vi "set-reporting-device.vi"(5 "ttl":i32, 6 "wait for reply (T)":bool=TRUE, 7 "device-name":string, 8 "error in":errorcluster, 9 "period-ms":i32, 10 "measurement-list":string[](array[string]), 11 "Module ID":i32=-1) -> (0 "error out":errorcluster, 1 "timed out?":bool, 2 "ack":bool)   [LabVIEW 2020, in "reporting-device.lvlib"]
doc: "_____\nCreated using DQMH Event Scripter 7.0.1.1316."
uses:
  reporting-device.lvlib
  set-reporting-device Argument--cluster.ctl
  set-reporting-device (Reply Payload)--cluster.ctl
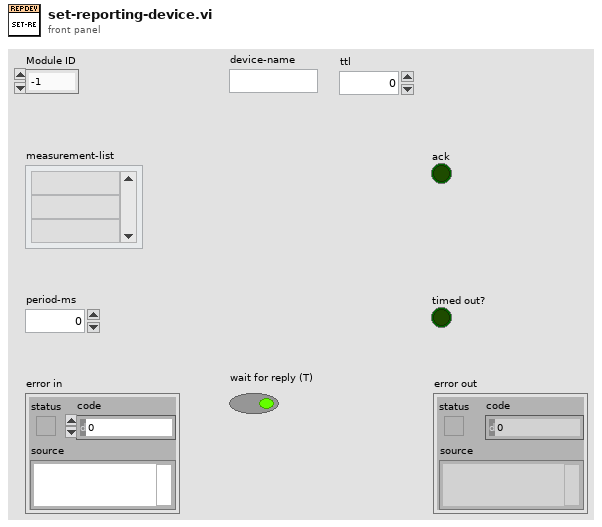
[diagram p1: front panel]
types:
  T1 = typedef "reporting-device.lvlib/set-reporting-device Argument--cluster.ctl" = cluster{"Module ID":i32, "measurement-list":string[], "period-ms":i32, "device-name":string, "ttl":i32, "Wait Notifier":refnum<notifier>, "wait for reply":bool}
  T2 = typedef "reporting-device.lvlib/Request Events--cluster.ctl" = cluster{"Stop Module":refnum<user-event>, "Show Panel":refnum<user-event>, "Hide Panel":refnum<user-event>, "Show Diagram":refnum<user-event>, "Get Module Execution Status":refnum<user-event>, "connect":refnum<user-event>, "start-publishing":refnum<user-event>, "set-reporting-device":refnum<user-event>}
  T3 = typedef "reporting-device.lvlib/set-reporting-device (Reply Payload)--cluster.ctl" = cluster{"Module ID":i32, "ack":bool, "error":errorcluster}
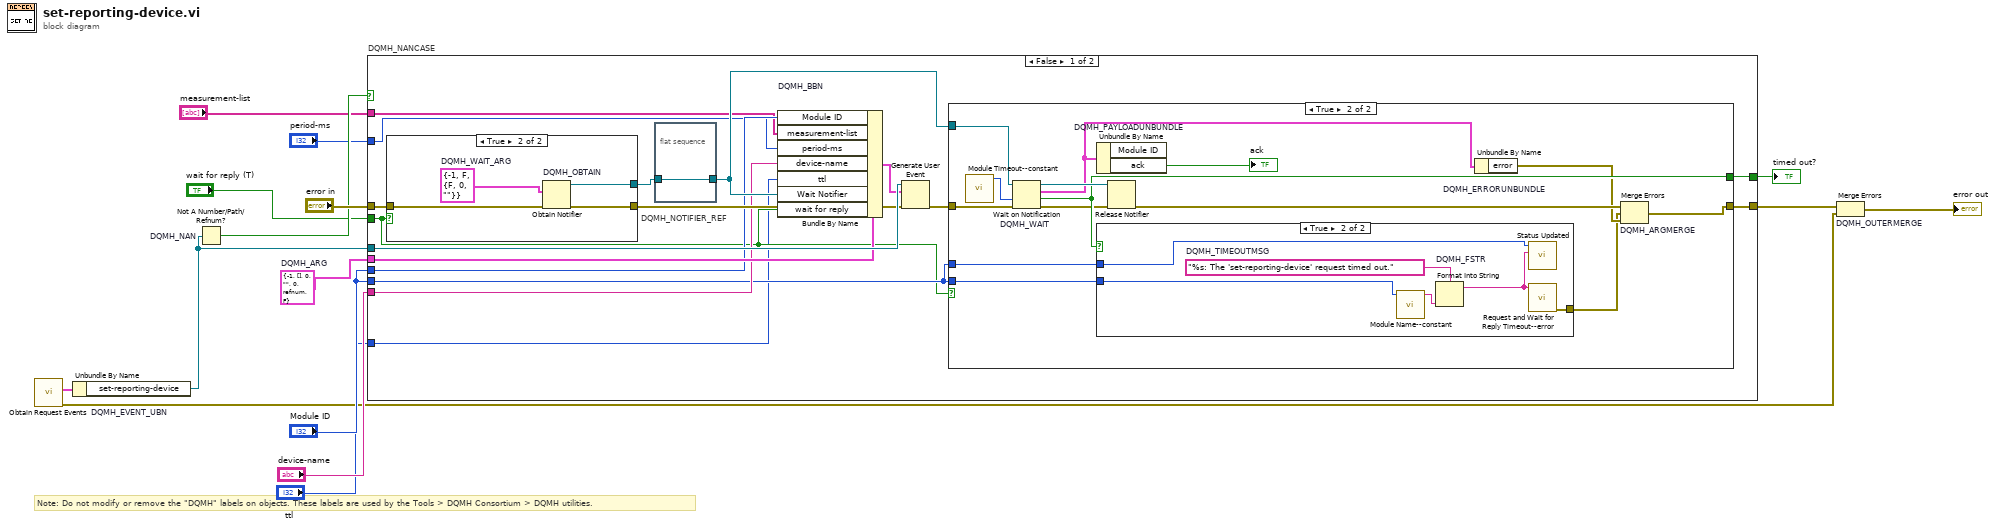
[diagram p0: block diagram]
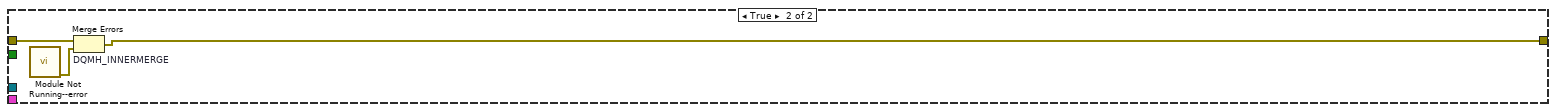
[diagram p5: hidden frame]
diagram:
  w2 = T1 {"Module ID"=-1, "measurement-list"=[], "period-ms"=0, "device-name"="", "ttl"=0, "Wait Notifier"=refnum, "wait for reply"=FALSE}  # DQMH_ARG
  # "Note: Do not modify or remove the \"DQMH\" labels on objects. These labels are used by the Tools > DQMH Consortium > DQMH utilities."
  n1 = call "Obtain Request Events.vi"() -> ("error out"=w4:errorcluster, "reporting-device Request Events"=w3:T2)  [unwired: 10 in]
  n2 = Unbundle By Name "DQMH_EVENT_UBN"(w3) -> ("set-reporting-device"=w13:refnum<user-event>)
  n3 = Not A Number/Path/Refnum? "DQMH_NAN"(number/path/refnum=w13) -> (NaN/Path/Refnum?=w12:bool)
  n4 = case "DQMH_NANCASE" shown="False" w12 {
    tunnel: "error in" -> [w32 w62]
    tunnel: w13 -> [w30 _]
    tunnel: [w27 w61] -> w10
    tunnel: [w28 _] -> w11
    tunnel: w2 -> [w23 _]
    tunnel: "Module ID" -> [w22 _]
    tunnel: "measurement-list" -> [w21 _]
    tunnel: "period-ms" -> [w20 _]
    tunnel: "device-name" -> [w19 _]
    tunnel: "Module ID" -> [w18 _]
    tunnel: "wait for reply (T)" -> [w17 _]
    tunnel: "ttl" -> [w16 _]
    frame False {
      n5 = case shown="True" w17 {
        tunnel: w32 -> [w55 w59]
        tunnel: [w55 w58] -> w29
        tunnel: [_ w56] -> w25
        frame False {
        }
        frame True {
          w57 = T3 {"Module ID"=-1, "ack"=FALSE, "error"={"status"=FALSE, "code"=0, "source"=""}}  # DQMH_WAIT_ARG
          n6 = Obtain Notifier "DQMH_OBTAIN"(notification data type=w57, error in (no error)=w59) -> (notifier out=w56:refnum<notifier>, error out=w58:errorcluster)  [unwired: 2 in, 1 out]
        }
      }
      n7 = flat-sequence "DQMH_NOTIFIER_REF" {
        tunnel: w25 -> [w33]
        tunnel: [w33] -> w24
        frame #0 {
        }
      }
      n8 = Bundle By Name "DQMH_BBN"(cluster=w23, "Module ID"=w22, "measurement-list"=w21, "period-ms"=w20, "device-name"=w19, "ttl"=w16, "Wait Notifier"=w24, "wait for reply"=w17) -> (w26:T1)
      n9 = Generate User Event(user event=w30, event data cluster=w26, error in=w29) -> (error out=w31:errorcluster)  [unwired: 1 in, 1 out]
      n10 = case shown="True" w17 {
        tunnel: w31 -> [w34 w48]
        tunnel: w24 -> [_ w47]
        tunnel: [_ w45] -> w28
        tunnel: [w34 w44] -> w27
        tunnel: w18 -> [_ w36]
        tunnel: w18 -> [_ w35]
        frame False {
        }
        frame True {
          n11 = call "Module Timeout--constant.vi"() -> ("Module Timeout"=w38:i32)  [unwired: 11 in]
          n12 = Wait on Notification "DQMH_WAIT"(notifier=w47, timeout in ms (-1)=w38, error in (no error)=w48) -> (notifier out=w46:refnum<notifier>, notification=w39:T3, timed out?=w45:bool, error out=w43:errorcluster)  [unwired: 1 in]
          n13 = Unbundle By Name "DQMH_PAYLOADUNBUNDLE"(w39) -> ("ack"=→"ack":bool)  [unwired: 1 out]
          n14 = case shown="True" w45 {
            tunnel: [_ w52] -> w40
            tunnel: w36 -> [_ w50]
            tunnel: w35 -> [_ w49]
            frame False {
            }
            frame True {
              w54 = "%s: The 'set-reporting-device' request timed out."  # DQMH_TIMEOUTMSG
              n15 = call "Module Name--constant.vi"("Module ID"=w49) -> ("Module Name"=w51:string)  [unwired: 10 in]
              n16 = Format Into String "DQMH_FSTR"(format string=w54, w51) -> (resulting string=w53:string)  [unwired: 2 in, 1 out]
              n17 = call "Status Updated.vi"("Status"=w53, "Module ID"=w50) -> ()  [unwired: 9 in, 1 out]
              n18 = call "Request and Wait for Reply Timeout--error.vi"("Error Message"=w53) -> ("error out"=w52:errorcluster)  [unwired: 10 in]
            }
          }
          n19 = Release Notifier(notifier=w46, error in (no error)=w43) -> (error out=w42:errorcluster)  [unwired: 1 in, 2 out]
          n20 = Unbundle By Name "DQMH_ERRORUNBUNDLE"(w39) -> ("error"=w41:errorcluster)
          n21 = Merge Errors "DQMH_ARGMERGE"(w42, w40, w41) -> (w44:errorcluster)
        }
      }
    }
    frame True {
      n22 = call "Module Not Running--error.vi"() -> ("error out"=w60:errorcluster)  [unwired: 11 in]
      n23 = Merge Errors "DQMH_INNERMERGE"(w62, w60) -> (w61:errorcluster)
    }
  }
  "timed out?" <- w11
  n24 = Merge Errors "DQMH_OUTERMERGE"(w10, w4) -> (→"error out":errorcluster)
